vi "Teleop.vi"(10 "Match Info":T1={"Autonomous Elapsed Seconds"=0.0, "TeleOp Elapsed Seconds"=0.0, "Disabled Elapsed Seconds"=0.0, "Visited Autonomous"=FALSE, "Visited TeleOp"=FALSE, "Visited Disabled"=FALSE, "Autonomous Settings"={"Autonomous Style"=enum."Independent", "VI Refnum"=refnum}}, 11 "Call Context":T2) -> ()   [LabVIEW 2015]
doc: "This VI is called for each TeleOp packet received from the DS where the robot is not disabled. It is often used to read from the joysticks and update I/O or to update setpoints for timed control loops. It should complete and return within 20 milliseconds or it may miss DS packets."
uses:
  <vilib>/Rock Robotics/WPI/DriverStation/WPI_DriverStationDerivedRobotMode.ctl
  <vilib>/Rock Robotics/WPI/DriverStation/WPI_DriverStationMatch Info.ctl
  <vilib>/Rock Robotics/WPI/Utilities/WPI_GetSetVariantRefNum.vi
  <vilib>/Rock Robotics/Network Tables/NT Write Boolean Array.vi
  <vilib>/Rock Robotics/Network Tables/NT Write Numeric Array.vi
  <vilib>/Rock Robotics/Network Tables/NT Write Number.vi
  <vilib>/Rock Robotics/Network Tables/NT Write Boolean.vi
  <vilib>/Rock Robotics/WPI/RobotDrive/WPI_RobotDriveArcadeDrive_Standard(NoSaturation).vi
  <vilib>/Rock Robotics/Network Tables/NT Read Number.vi
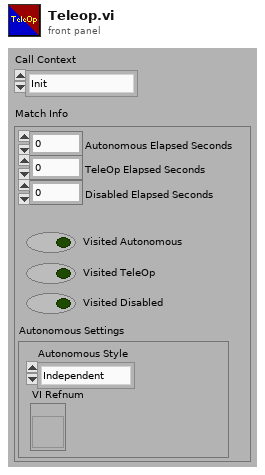
[diagram p1: front panel]
types:
  T1 = typedef "WPI_DriverStationMatch Info.ctl" = cluster{"Autonomous Elapsed Seconds":dbl, "TeleOp Elapsed Seconds":dbl, "Disabled Elapsed Seconds":dbl, "Visited Autonomous":bool, "Visited TeleOp":bool, "Visited Disabled":bool, "Autonomous Settings":cluster{"Autonomous Style":enum16{"Iterative", "Independent"}, "VI Refnum":refnum<vi>}}
  T2 = typedef "WPI_DriverStationDerivedRobotMode.ctl" = enum16{"Init", "Execute", "Stop"}
  T3 = typedef "WPI_GyroDevRef.ctl" = cluster{"DevStatus":errorcluster, "Analog Channel":T4, "Offset":dbl, "Gain (VoltsPerDegree/Second)":dbl, "Gyro Type":enum16{"Analog", "XRS450"}, "Handle":i32, "SPI Bus":T5, "Device Found":bool, "Sample Rate":dbl, "Calibrate On Open":bool}
  T4 = typedef "FPGA_AIChannel.ctl" = enum8{"AI 0", "AI 1", "AI 2", "AI 3", "AI MXP 0", "AI MXP 1", "AI MXP 2", "AI MXP 3", "Invalid"}
  T5 = typedef "spi_bus.ctl" = enum16{"SPI On-Board, CS0", "SPI On-Board, CS1", "SPI On-Board, CS2", "SPI On-Board, CS3", "SPI MXP", "Invalid"}
  T6 = typedef "WPI_JoystickDevRef.ctl" = cluster{"Device":T7}
  T7 = typedef "WPI_JoystickDeviceEnum.ctl" = enum16{"USB 0", "USB 1", "USB 2", "USB 3", "USB 4", "USB 5"}
  T8 = cluster{"POVs[0]":i16, "POVs[1]":i16, "POVs[2]":i16, "POVs[3]":i16, "POVs[4]":i16, "POVs[5]":i16, "POVs[6]":i16, "POVs[7]":i16, "POVs[8]":i16}
  T9 = typedef "WPI_AnalogChannelDevRef.ctl" = cluster{"DevStatus":errorcluster, "Analog Channel":T4}
  T10 = typedef "WPI_ServoDeviceRef.ctl" = cluster{"DeviceStatus":errorcluster, "PWM Channel":T11, "DeadBand":T12}
  T11 = typedef "FPGA_DIOPWMChannel.ctl" = enum8{"PWM 0", "PWM 1", "PWM 2", "PWM 3", "PWM 4", "PWM 5", "PWM 6", "PWM 7", "PWM 8", "PWM 9", "PWM MXP 0", "PWM MXP 1", "PWM MXP 2", "PWM MXP 3", "PWM MXP 4", "PWM MXP 5", "PWM MXP 6", "PWM MXP 7", "PWM MXP 8", "PWM MXP 9", "Invalid"}
  T12 = typedef "WPI_PWMDeadband.ctl" = cluster{"Name":string, "maxPositivePwm":i32, "minPositivePwm":i32, "centerPwm":i32, "maxNegativePwm":i32, "minNegativePwm":i32, "angularRange":u16}
  T13 = typedef "WPI_RobotDriveDevRef.ctl" = cluster{"DevStatus":errorcluster, "Motors[]":T14[], "Square Inputs":bool, "Max Output":dbl}
  T14 = typedef "WPI_MotorControlDeviceRef.ctl" = cluster{"DeviceStatus":errorcluster, "Type":T15, "PWM":cluster{"PWM Channel":T11, "DeadBand":T12}, "CAN":cluster{"Device Number":u8, "Control Mode":T16, "Semaphore":T17, "Max Vout":dbl, "TalonSRX Control Mode":T18}, "Invert":bool}
  T15 = typedef "WPI_MotorControlType.ctl" = enum16{"PWM", "CAN", "CANTalonSRX"}
  T16 = typedef "WPI_CANJaguar_ControlMode.ctl" = enum8{"Percent VBus", "Current", "Speed", "Position", "Voltage"}
  T17 = typedef "Semaphore RefNum" = refnum<k1>
  T18 = typedef "WPI_CANTalonSRX_APIControlMode.ctl" = enum8{"Percent VBus", "Speed", "Position", "Slave", "Unchanged / Invalid", "Voltage Compensation", "Current", "Motion Profile"}
  T19 = cluster{"Buttons[0]":bool, "Buttons[1]":bool, "Buttons[2]":bool, "Buttons[3]":bool, "Buttons[4]":bool, "Buttons[5]":bool, "Buttons[6]":bool, "Buttons[7]":bool, "Buttons[8]":bool}
  T20 = typedef "WPI_DigitalInputDevRef.ctl" = cluster{"DevStatus":errorcluster, "DIO Channel":T21}
  T21 = typedef "FPGA_DIOChannel.ctl" = enum8{"DIO 0", "DIO 1", "DIO 2", "DIO 3", "DIO 4", "DIO 5", "DIO 6", "DIO 7", "DIO 8", "DIO 9", "DIO MXP 0", "DIO MXP 1", "DIO MXP 2", "DIO MXP 3", "DIO MXP 4", "DIO MXP 5", "DIO MXP 6", "DIO MXP 7", "DIO MXP 8", "DIO MXP 9", "DIO MXP 10", "DIO MXP 11", "DIO MXP 12", "DIO MXP 13", "DIO MXP 14", "DIO MXP 15", "Invalid"}
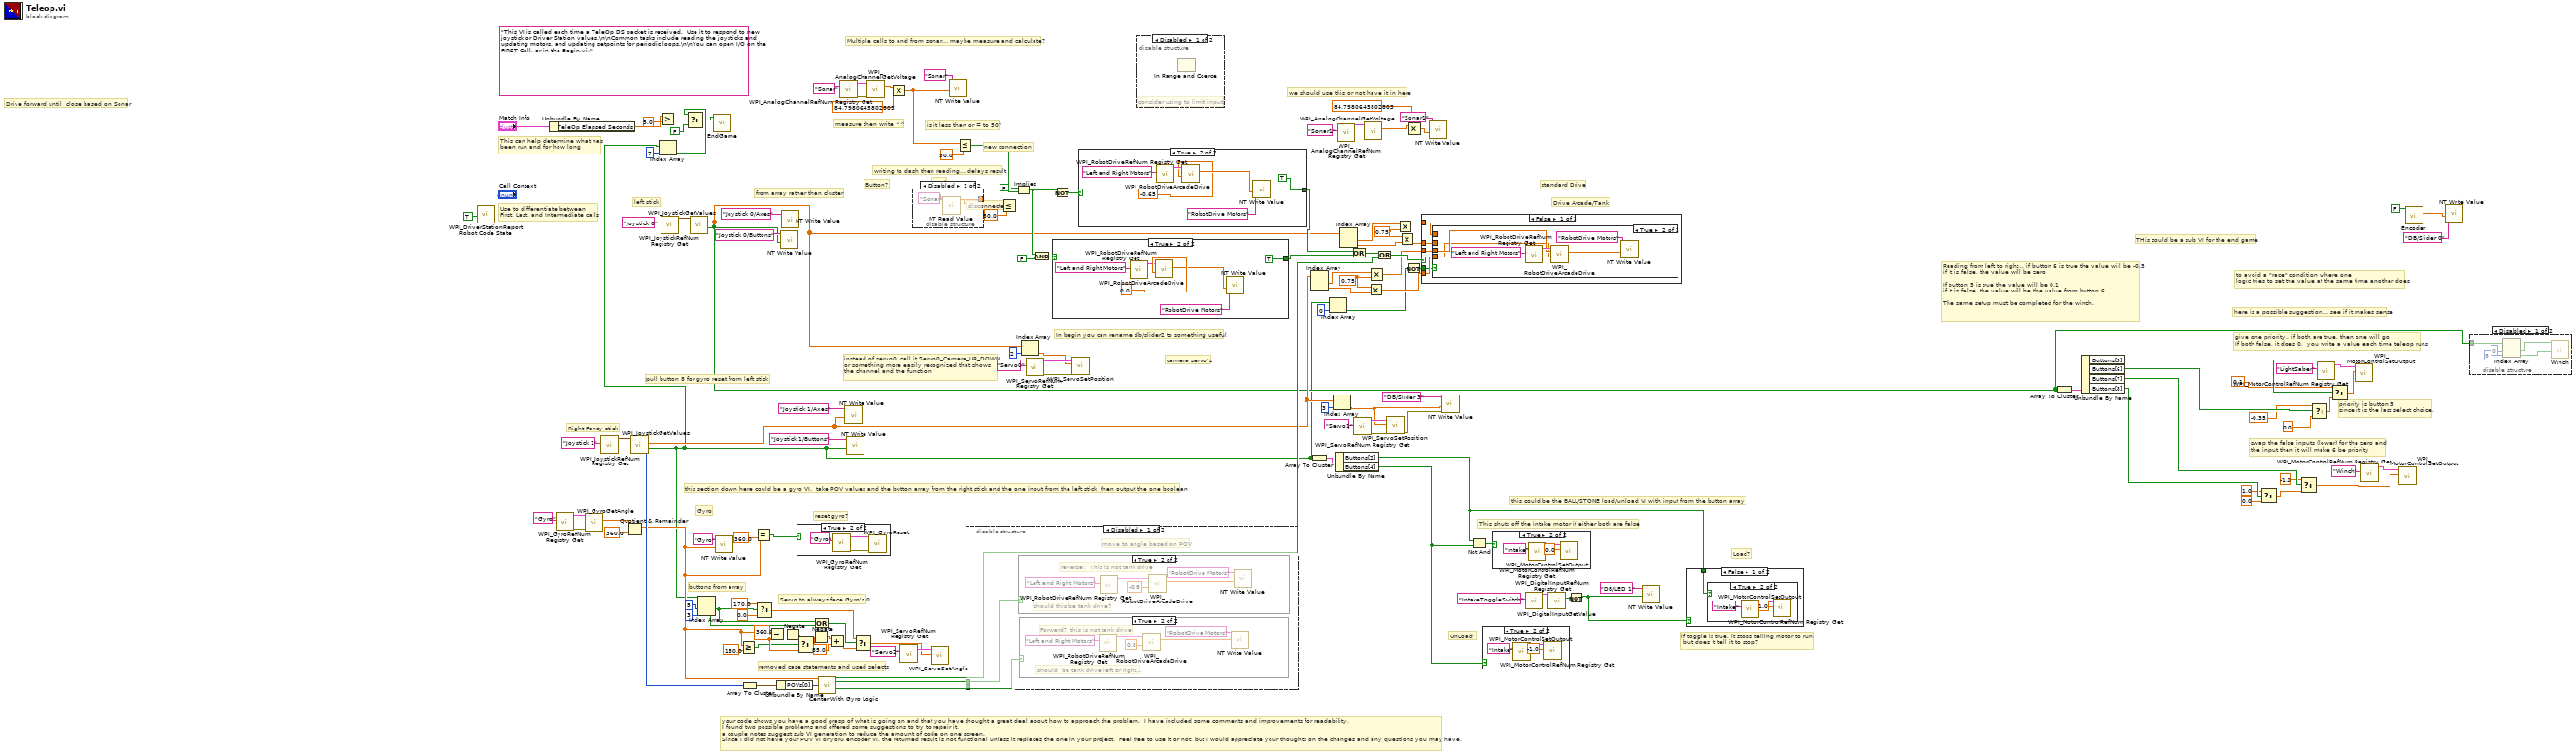
[diagram p0: block diagram]
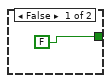
[diagram p11: hidden frame]
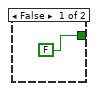
[diagram p12: hidden frame]
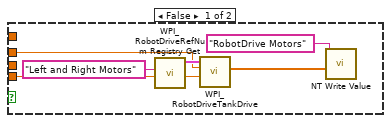
[diagram p14: hidden frame]
diagram:
  w61 = 0.75
  w75 = 0.75
  (unwired) "This VI is called each time a TeleOp DS packet is received.  Use it to respond to new joystick or Driver Station values.\n\nCommon tasks include reading the joysticks and updating motors, and updating setpoints for periodic loops.\n\nYou can open I/O on the FIRST Call, or in the Begin.vi."
  # "swap the false inputs (lower) for the zero and\nthe input then it will make 6 be priority"
  # "priority is button 5\nsince it is the last select choice."
  # "give one priority.. if both are true, then one will go\nIf both false, it does 0.  you write a value each time teleop runs"
  # "Reading from left to right... if button 6 is true the value will be -0.5\nif it is false, the value will be zero\n\nIf button 5 is true the value will be 0.1\nif it is false, the value will be the value from button 6.\n\nThe same setup must be completed for the winch."
  # "to avoid a \"race\" condition where one \nlogic tries to set the value at the same time another does"
  # "here is a possible suggestion... see if it makes sense"
  # "we should use this or not have it in here"
  # "THis could be a sub VI for the end game"
  # "your code shows you have a good grasp of what is going on and that you have thought a great deal about how to approach the problem.  I have included some comments and improvements for readability.\nI found two possible problems and offered some suggestions to try to repair it. \na couple notes suggest sub VI generation to reduce the amount of code on one screen.\nSince I did not have your POV VI or yoru encoder VI, the returned result is not functional unless it replaces the one in your project.  Feel free to use it or not, but I would appreciate your thoughts on the changes and any questions you may have."
  # "if toggle is true, it stops telling motor to run,\n but does it tell it to stop?"
  # "this could be the BALL/STONE load/unload VI with input from the button array"
  # "this section down here could be a gyro VI.  take POV values and the button array from the right stick and the one input from the left stick  then output the one boolean"
  # "This shuts off the intake motor if either both are false"
  # "Load?"
  # "UnLoad?"
  # "pull button 8 for gyro reset from left stick"
  # "reset gyro?"
  # "Gyro"
  # "removed case statements and used selects"
  # "buttons from array"
  # "Right Fancy stick"
  # "left stick"
  # "from array rather than cluster"
  # "new connection"
  # "disconnected"
  # "read"
  # "measure then write ^^"
  # "writing to dash then reading... delays result"
  # "is it less than or = to 50?"
  # "Multiple calls to and from sonar... maybe measure and calculate?"
  # "Button?"
  # "standard Drive"
  # "instead of servo0, call it Servo0_Camera_UP_DOWN\nor something more easily recognized that shows\nthe channel and the function"
  # "In begin you can rename db/slider2 to something useful"
  # "Servo to always face Gyro's 0"
  # "camera servo's"
  # "Drive Arcade/Tank"
  # "Drive forward until  close based on Sonar"
  # "Use to differentiate between\nFirst, Last, and Intermediate calls"
  # "This can help determine what has\nbeen run and for how long"
  n1 = call <vilib>:"WPI_DriverStationReport Robot Code State.vi"("TeleOp"=TRUE ("Autonomous")) -> ()  [unwired: 10 in, 1 out]
  n2 = Unbundle By Name("Match Info") -> ("TeleOp Elapsed Seconds"=w33:dbl)
  n3 = call <vilib>:"WPI_GyroRefNum Registry Get.vi"("refnum name"="Gyro") -> ("error out"=w42:errorcluster, "GyroDevRef"=w123:T3)  [unwired: 9 in]
  n4 = call <vilib>:"WPI_GyroGetAngle.vi"("error in"=w42, "GyroDevRef"=w123) -> ("Angle"=w118:dbl)  [unwired: 5 in, 4 out]
  n5 = call <vilib>:"WPI_JoystickRefNum Registry Get.vi"("refnum name"="Joystick 1") -> ("JoystickDevRef"=w131:T6)  [unwired: 1 in, 9 out]
  n6 = Quotient & Remainder(x=w118, y=360.0) -> (x-y*floor(x/y)=w100:dbl)  [unwired: 1 out]
  n7 = call <vilib>:"WPI_JoystickGetValues.vi"("JoystickDevRef"=w131) -> ("Buttons"=w3:bool[], "Axes"=w68:dbl[], "POVs"=w106:i16[])  [unwired: 6 in, 2 out]
  n8 = Index Array(array=w3, index=7) -> (element=w10:bool)
  n9 = Greater?(x=w33, y=5.0) -> (0:w11:bool)
  n10 = call <vilib>:"WPI_JoystickRefNum Registry Get.vi"("refnum name"="Joystick 0") -> ("JoystickDevRef"=w135:T6)  [unwired: 1 in, 9 out]
  n11 = Select(t=w10, s=w11, f=FALSE) -> (s? t:f=w8:bool)
  n12 = call <vilib>:"WPI_JoystickGetValues.vi"("JoystickDevRef"=w135) -> ("Buttons"=w32:bool[], "Axes"=w71:dbl[])  [unwired: 6 in, 3 out]
  n13 = Index Array(array=w3, index #1=5 ("index"), index #2=3 ("index")) -> (element #1=w41:bool, element #2=w40:bool)
  n14 = call "EndGame.vi"("End Game?"=w8) -> ()  [unwired: 11 in]
  n15 = call-poly <vilib>:"NT Write Value.vi"("Numeric"=w100, "Name"="Gyro") -> ()  [unwired: 9 in, 1 out]
  n16 = Greater Or Equal?(x=w100, y=180.0) -> (x >= y?=w49:bool)
  n17 = Array To Cluster(array=w106) -> (cluster=w109:T8)
  n18 = Equal?(x=w100, y=360.0) -> (x = y?=w14:bool)
  n19 = Select(t=170.0, s=w41, f=0.0) -> (s? t:f=w45:dbl)
  n20 = Subtract(x=360.0, y=w100) -> (x-y=w51:dbl)
  n21 = Unbundle By Name(w109) -> ("POVs[0]"=w108:i16)
  n22 = call-poly <vilib>:"NT Write Value.vi"("Boolean Array"=w32, "Name"="Joystick 0/Buttons") -> ()  [unwired: 9 in, 1 out]
  n23 = call-poly <vilib>:"NT Write Value.vi"("Numeric Array"=w71, "Name"="Joystick 0/Axes") -> ()  [unwired: 9 in, 1 out]
  n24 = Negate(x=w51) -> (-x=w55:dbl)
  n25 = case shown="True" w14 {
    frame False {
    }
    frame True {
      n26 = call <vilib>:"WPI_GyroRefNum Registry Get.vi"("refnum name"="Gyro") -> ("error out"=w139:errorcluster, "GyroDevRef"=w141:T3)  [unwired: 9 in]
      n27 = call <vilib>:"WPI_GyroReset.vi"("error in"=w139, "GyroDevRef"=w141) -> ()  [unwired: 8 in, 2 out]
    }
  }
  n28 = Select(t=w55, s=w49, f=w100) -> (s? t:f=w50:dbl)
  n29 = Negate(x=w50) -> (-x=w54:dbl)
  n30 = Or(x=w41, y=w40) -> (x .or. y?=w46:bool)
  n31 = call "Center With Gyro Logic.vi"("Angle"=w100, "Face Where?"=w108) -> ("Disable Drive"=w116:bool, "Too Far to the Right"=w121:bool, "Too Far to the Left"=w120:bool)  [unwired: 11 in]
  n32 = Add(x=w54, y=85.0) -> (x+y=w48:dbl)
  n33 = call <vilib>:"WPI_AnalogChannelRefNum Registry Get.vi"("refnum name"="Sonar") -> ("error out"=w63:errorcluster, "AIDeviceRef"=w104:T9)  [unwired: 9 in]
  n34 = call-poly <vilib>:"NT Write Value.vi"("Numeric Array"=w68, "Name"="Joystick 1/Axes") -> ()  [unwired: 9 in, 1 out]
  n35 = call-poly <vilib>:"NT Write Value.vi"("Boolean Array"=w3, "Name"="Joystick 1/Buttons") -> ()  [unwired: 9 in, 1 out]
  n36 = Select(t=w45, s=w46, f=w48) -> (s? t:f=w47:dbl)
  n37 = call <vilib>:"WPI_AnalogChannelGetVoltage.vi"("error in (no error)"=w63, "AIDeviceRef"=w104) -> ("Voltage"=w102:dbl)  [unwired: 7 in, 2 out]
  n38 = Multiply(x=w102, y=84.7980645802803) -> (x*y=w64:dbl)
  n39 = call <vilib>:"WPI_ServoRefNum Registry Get.vi"("refnum name"="Servo2") -> ("ServoDeviceRef"=w59:T10)  [unwired: 9 in, 1 out]
  n40 = disable-structure shown="Disabled" {
    disable-tunnel: [w143 _] -> w98
    frame Disabled {
      n41 = call-poly <vilib>:"NT Read Value.vi"("Name"="Sonar") -> ("Numeric"=w143:dbl)  [unwired: 9 in, 1 out]
    }
    frame Enabled {
    }
  }
  n42 = call <vilib>:"WPI_ServoSetAngle.vi"("Angle"=w47, "ServoDeviceRef"=w59) -> ()  [unwired: 8 in, 2 out]
  n43 = call-poly <vilib>:"NT Write Value.vi"("Numeric"=w64, "Name"="Sonar") -> ()  [unwired: 9 in, 1 out]
  n44 = Less Or Equal?(x=w64, y=50.0) -> (x <= y?=w65:bool)
  n45 = disable-structure shown="Disabled" {
    disable-tunnel: w121 -> [w145 _]
    disable-tunnel: w120 -> [w144 _]
    frame Disabled {
      # "move to angle based on POV"
      n46 = case shown="True" w145 {
        frame False {
        }
        frame True {
          # "should this be tank drive?"
          # "reverse?  This is not tank drive"
          n47 = call <vilib>:"WPI_RobotDriveRefNum Registry Get.vi"("refnum name"="Left and Right Motors") -> ("RobotDriveDevRef"=w153:T13)  [unwired: 9 in, 1 out]
          n48 = call-poly <vilib>:"WPI_RobotDriveArcadeDrive.vi"("X axis value"=-0.8, "RobotDriveDevRef"=w153) -> ("Motor Values"=w154:dbl[])  [unwired: 7 in, 2 out]
          n49 = call-poly <vilib>:"NT Write Value.vi"("Numeric Array"=w154, "Name"="RobotDrive Motors") -> ()  [unwired: 9 in, 1 out]
        }
      }
      n50 = case shown="True" w144 {
        frame False {
        }
        frame True {
          # "should  be tank drive left or right..."
          # "Forward?  this is not tank drive"
          n51 = call <vilib>:"WPI_RobotDriveRefNum Registry Get.vi"("refnum name"="Left and Right Motors") -> ("RobotDriveDevRef"=w148:T13)  [unwired: 9 in, 1 out]
          n52 = call-poly <vilib>:"WPI_RobotDriveArcadeDrive.vi"("X axis value"=0.8, "RobotDriveDevRef"=w148) -> ("Motor Values"=w149:dbl[])  [unwired: 7 in, 2 out]
          n53 = call-poly <vilib>:"NT Write Value.vi"("Numeric Array"=w149, "Name"="RobotDrive Motors") -> ()  [unwired: 9 in, 1 out]
        }
      }
    }
    frame Enabled {
    }
  }
  n54 = Less Or Equal?(x=w98, y=50.0) -> ()  [unwired: 1 out]
  n55 = Implies(1:w65, 2:FALSE ("x")) -> (0:w93:bool)
  n56 = Index Array(array=w71, index=2) -> (element=w72:dbl)
  n57 = call <vilib>:"WPI_ServoRefNum Registry Get.vi"("refnum name"="Servo0") -> ("error out"=w76:errorcluster, "ServoDeviceRef"=w113:T10)  [unwired: 9 in]
  n58 = And(x=w93, y=FALSE) -> (x .and. y?=w94:bool)
  n59 = case shown="True" w94 {
    tunnel: [FALSE TRUE] -> w91
    frame False {
    }
    frame True {
      n60 = call <vilib>:"WPI_RobotDriveRefNum Registry Get.vi"("refnum name"="Left and Right Motors") -> ("RobotDriveDevRef"=w160:T13)  [unwired: 9 in, 1 out]
      n61 = call-poly <vilib>:"WPI_RobotDriveArcadeDrive.vi"("Y axis value"=0.0 ("X axis value"), "RobotDriveDevRef"=w160) -> ("Motor Values"=w159:dbl[])  [unwired: 7 in, 2 out]
      n62 = call-poly <vilib>:"NT Write Value.vi"("Numeric Array"=w159, "Name"="RobotDrive Motors") -> ()  [unwired: 9 in, 1 out]
    }
  }
  n63 = Not(x=w93) -> (.not. x?=w95:bool)
  n64 = call <vilib>:"WPI_ServoSetPosition.vi"("error in (no error)"=w76, "Position"=w72, "ServoDeviceRef"=w113) -> ()  [unwired: 7 in, 2 out]
  n65 = case shown="True" w95 {
    tunnel: [FALSE TRUE] -> w96
    frame False {
    }
    frame True {
      n66 = call <vilib>:"WPI_RobotDriveRefNum Registry Get.vi"("refnum name"="Left and Right Motors") -> ("RobotDriveDevRef"=w167:T13)  [unwired: 9 in, 1 out]
      n67 = call-poly <vilib>:"WPI_RobotDriveArcadeDrive.vi"("Y axis value"=-0.65 ("X axis value"), "RobotDriveDevRef"=w167) -> ("Motor Values"=w168:dbl[])  [unwired: 7 in, 2 out]
      n68 = call-poly <vilib>:"NT Write Value.vi"("Numeric Array"=w168, "Name"="RobotDrive Motors") -> ()  [unwired: 9 in, 1 out]
    }
  }
  n69 = disable-structure shown="Disabled" {
    frame Disabled {
      # "consider using to limit input"
      n70 = In Range and Coerce() -> ()  [unwired: 3 in, 2 out]
    }
    frame Enabled {
    }
  }
  n71 = Index Array(array=w68) -> (element #1=w128:dbl, element #2=w62:dbl)  [unwired: 2 in]
  n72 = Array To Cluster(array=w3) -> (cluster=w125:T19)
  n73 = Index Array(array=w3, index=0) -> (element=w2:bool)
  n74 = Index Array(array=w68, index=3) -> (element=w69:dbl)
  n75 = Unbundle By Name(w125) -> ("Buttons[2]"=w39:bool, "Buttons[4]"=w38:bool)
  n76 = call <vilib>:"WPI_AnalogChannelRefNum Registry Get.vi"("refnum name"="Sonar1") -> ("AIDeviceRef"=w89:T9)  [unwired: 9 in, 1 out]
  n77 = Index Array(array=w71) -> (element #1=w127:dbl, element #2=w74:dbl)  [unwired: 2 in]
  n78 = Or(x=w96, y=w91) -> (x .or. y?=w92:bool)
  n79 = call <vilib>:"WPI_ServoRefNum Registry Get.vi"("refnum name"="Servo1") -> ("error out"=w78:errorcluster, "ServoDeviceRef"=w111:T10)  [unwired: 9 in]
  n80 = call <vilib>:"WPI_AnalogChannelGetVoltage.vi"("AIDeviceRef"=w89) -> ("Voltage"=w87:dbl)  [unwired: 8 in, 2 out]
  n81 = Multiply(x=w61, y=w62) -> (x*y=w115:dbl)
  n82 = Multiply(x=w128, y=w61) -> (x*y=w7:dbl)
  n83 = Or(x=w92, y=w116) -> (x .or. y?=w99:bool)
  n84 = call <vilib>:"WPI_ServoSetPosition.vi"("error in (no error)"=w78, "Position"=w69, "ServoDeviceRef"=w111) -> ("error out"=w77:errorcluster)  [unwired: 7 in, 1 out]
  n85 = Multiply(x=w127, y=w75) -> (x*y=w119:dbl)
  n86 = Multiply(x=w75, y=w74) -> (x*y=w70:dbl)
  n87 = Not(x=w2) -> (.not. x?=w6:bool)
  n88 = Multiply(x=w87, y=84.7980645802803) -> (x*y=w86:dbl)
  n89 = case shown="False" w99 {
    tunnel: w70 -> [w172 _]
    tunnel: w115 -> [w174 _]
    tunnel: w119 -> [w171 _]
    tunnel: w6 -> [w173 _]
    tunnel: w7 -> [w170 _]
    frame False {
      n90 = case shown="True" w173 {
        tunnel: w172 -> [w176 _]
        tunnel: w174 -> [w175 w181]
        tunnel: w171 -> [_ _]
        tunnel: w170 -> [_ w182]
        frame False {
          n91 = call <vilib>:"WPI_RobotDriveRefNum Registry Get.vi"("refnum name"="Left and Right Motors") -> ("RobotDriveDevRef"=w180:T13)  [unwired: 9 in, 1 out]
          n92 = call <vilib>:"WPI_RobotDriveTankDrive.vi"("Right axis value"=w175, "Left axis value"=w176, "RobotDriveDevRef"=w180) -> ("Motor Values"=w178:dbl[])  [unwired: 6 in, 2 out]
          n93 = call-poly <vilib>:"NT Write Value.vi"("Numeric Array"=w178, "Name"="RobotDrive Motors") -> ()  [unwired: 9 in, 1 out]
        }
        frame True {
          n94 = call <vilib>:"WPI_RobotDriveRefNum Registry Get.vi"("refnum name"="Left and Right Motors") -> ("RobotDriveDevRef"=w184:T13)  [unwired: 9 in, 1 out]
          n95 = call-poly <vilib>:"WPI_RobotDriveArcadeDrive.vi"("Y axis value"=w181, "X axis value"=w182, "RobotDriveDevRef"=w184) -> ("Motor Values"=w185:dbl[])  [unwired: 6 in, 2 out]
          n96 = call-poly <vilib>:"NT Write Value.vi"("Numeric Array"=w185, "Name"="RobotDrive Motors") -> ()  [unwired: 9 in, 1 out]
        }
      }
    }
    frame True {
    }
  }
  n97 = call-poly <vilib>:"NT Write Value.vi"("Numeric"=w86, "Name"="Sonar1") -> ()  [unwired: 9 in, 1 out]
  n98 = call-poly <vilib>:"NT Write Value.vi"("error in"=w77, "Numeric"=w69, "Name"="DB/Slider 3") -> ()  [unwired: 8 in, 1 out]
  n99 = Not And(1:w38, 2:w39) -> (0:w81:bool)
  n100 = case shown="True" w38 {
    frame False {
    }
    frame True {
      n101 = call <vilib>:"WPI_MotorControlRefNum Registry Get.vi"("refnum name"="Intake") -> ("MotorControlDevRef"=w188:T14)  [unwired: 9 in, 1 out]
      n102 = call <vilib>:"WPI_MotorControlSetOutput.vi"("Output"=-1.0, "MotorControlDevRef"=w188) -> ()  [unwired: 7 in, 3 out]
    }
  }
  n103 = case shown="True" w81 {
    frame False {
    }
    frame True {
      n104 = call <vilib>:"WPI_MotorControlRefNum Registry Get.vi"("refnum name"="Intake") -> ("MotorControlDevRef"=w191:T14)  [unwired: 9 in, 1 out]
      n105 = call <vilib>:"WPI_MotorControlSetOutput.vi"("Output"=0.0, "MotorControlDevRef"=w191) -> ()  [unwired: 7 in, 3 out]
    }
  }
  n106 = call <vilib>:"WPI_DigitalInputRefNum Registry Get.vi"("refnum name"="IntakeToggleSwitch") -> ("DigitalInputDevRef"=w84:T20)  [unwired: 9 in, 1 out]
  n107 = call <vilib>:"WPI_DigitalInputGetValue.vi"("DigitalInputDevRef"=w84) -> ("Value"=w82:bool)  [unwired: 8 in, 2 out]
  n108 = Not(x=w82) -> (.not. x?=w79:bool)
  n109 = call-poly <vilib>:"NT Write Value.vi"("Boolean"=w79, "Name"="DB/LED 1") -> ()  [unwired: 9 in, 1 out]
  n110 = case shown="False" w79 {
    tunnel: w39 -> [w193 _]
    frame False {
      n111 = case shown="True" w193 {
        frame False {
        }
        frame True {
          n112 = call <vilib>:"WPI_MotorControlRefNum Registry Get.vi"("refnum name"="Intake") -> ("MotorControlDevRef"=w195:T14)  [unwired: 9 in, 1 out]
          n113 = call <vilib>:"WPI_MotorControlSetOutput.vi"("Output"=1.0, "MotorControlDevRef"=w195) -> ()  [unwired: 7 in, 3 out]
        }
      }
    }
    frame True {
    }
  }
  n114 = Array To Cluster(array=w32) -> (cluster=w126:T19)
  n115 = Unbundle By Name(w126) -> ("Buttons[5]"=w37:bool, "Buttons[6]"=w36:bool, "Buttons[7]"=w35:bool, "Buttons[8]"=w34:bool)
  n116 = Select(t=1.0, s=w34, f=0.0) -> (s? t:f=w21:dbl)
  n117 = Select(t=-1.0, s=w35, f=w21) -> (s? t:f=w15:dbl)
  n118 = Select(t=-0.35 ("Output"), s=w36, f=0.0 ("Output")) -> (s? t:f=w25:dbl)
  n119 = call <vilib>:"WPI_MotorControlRefNum Registry Get.vi"("refnum name"="LightSaber") -> ("MotorControlDevRef"=w31:T14)  [unwired: 9 in, 1 out]
  n120 = Select(t=0.1 ("Output"), s=w37, f=w25) -> (s? t:f=w26:dbl)
  n121 = call <vilib>:"WPI_MotorControlSetOutput.vi"("Output"=w26, "MotorControlDevRef"=w31) -> ()  [unwired: 7 in, 3 out]
  n122 = call <vilib>:"WPI_MotorControlRefNum Registry Get.vi"("refnum name"="Winch") -> ("MotorControlDevRef"=w17:T14)  [unwired: 9 in, 1 out]
  n123 = call <vilib>:"WPI_MotorControlSetOutput.vi"("Output"=w15, "MotorControlDevRef"=w17) -> ()  [unwired: 7 in, 3 out]
  n124 = call "Encoder.vi"("Reset Encoder?"=FALSE) -> ("revolutions"=w23:dbl)  [unwired: 7 in, 3 out]
  n125 = call-poly <vilib>:"NT Write Value.vi"("Numeric"=w23, "Name"="DB/Slider 0") -> ()  [unwired: 9 in, 1 out]
  n126 = disable-structure shown="Disabled" {
    disable-tunnel: w32 -> [w201 _]
    frame Disabled {
      n127 = Index Array(array=w201, index #1=0 ("index"), index #2=8 ("index")) -> (element #1=w199:bool, element #2=w197:bool)
      n128 = call "Winch.vi"("Reset Encoder?"=w197, "Run Winch"=w199) -> ()  [unwired: 10 in]
    }
    frame Enabled {
    }
  }
